vi "AcquisitionMVF_Reentrent.vi"(1 "cam conneced":bool, 4 "Numeric":i32, 5 "fake image type":enum16{"moving", "picture", "noise"}(ring), 6 "error in":errorcluster, 7 "Session":T2, 9 "Image Rev":T1) -> (0 "camera error":errorcluster, 2 "Image Dst Out":T1, 3 "Acquisition OK?":bool, 8 "time":u32)   [LabVIEW 2011]
uses:
  IMAQ Image.ctl
  IMAQdx.ctl
  NI_Vision_Development_Module.lvlib
  NI_Vision_Acquisition_Software.lvlib
  NI_AALBase.lvlib
panel:
  out "Image Out":T1
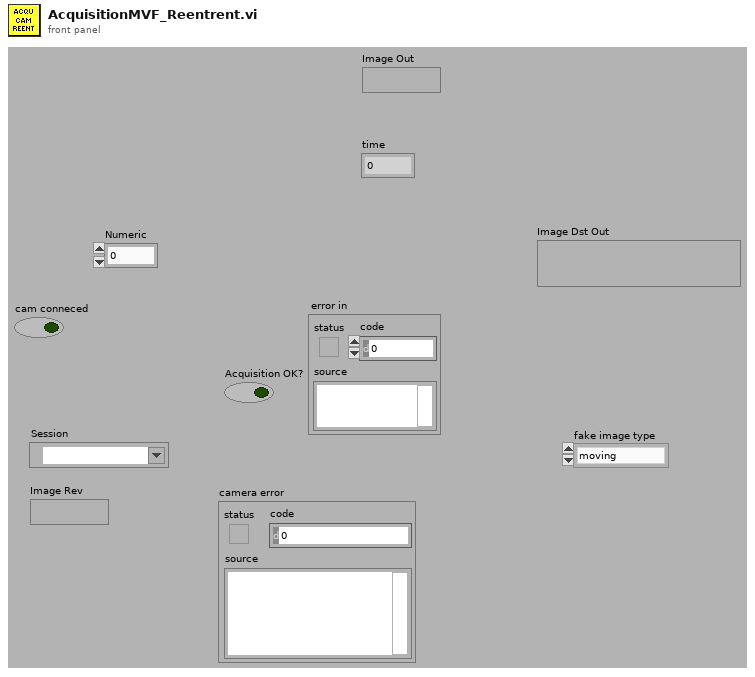
[diagram p1: front panel]
types:
  T1 = typedef "IMAQ Image.ctl" = refnum<image>
  T2 = typedef "IMAQdx.ctl" = refnum<k21>
  T3 = cluster{"Desired Font (Application)":enum16{"User-specified Font", "Application Font", "System Font", "Dialog Font"}, "[User-specified Font]":cluster{"Font Name":string, "Size":i16, "Strikeout?":bool, "Italic?":bool, "Underline?":bool, "Outline?":bool, "Shadow?":bool, "Bold?":bool, "Rotation Angle":dbl}, "Horizontal Alignment":i16, "Vertical Alignment":i16}
  T4 = typedef "Image Type" = u32
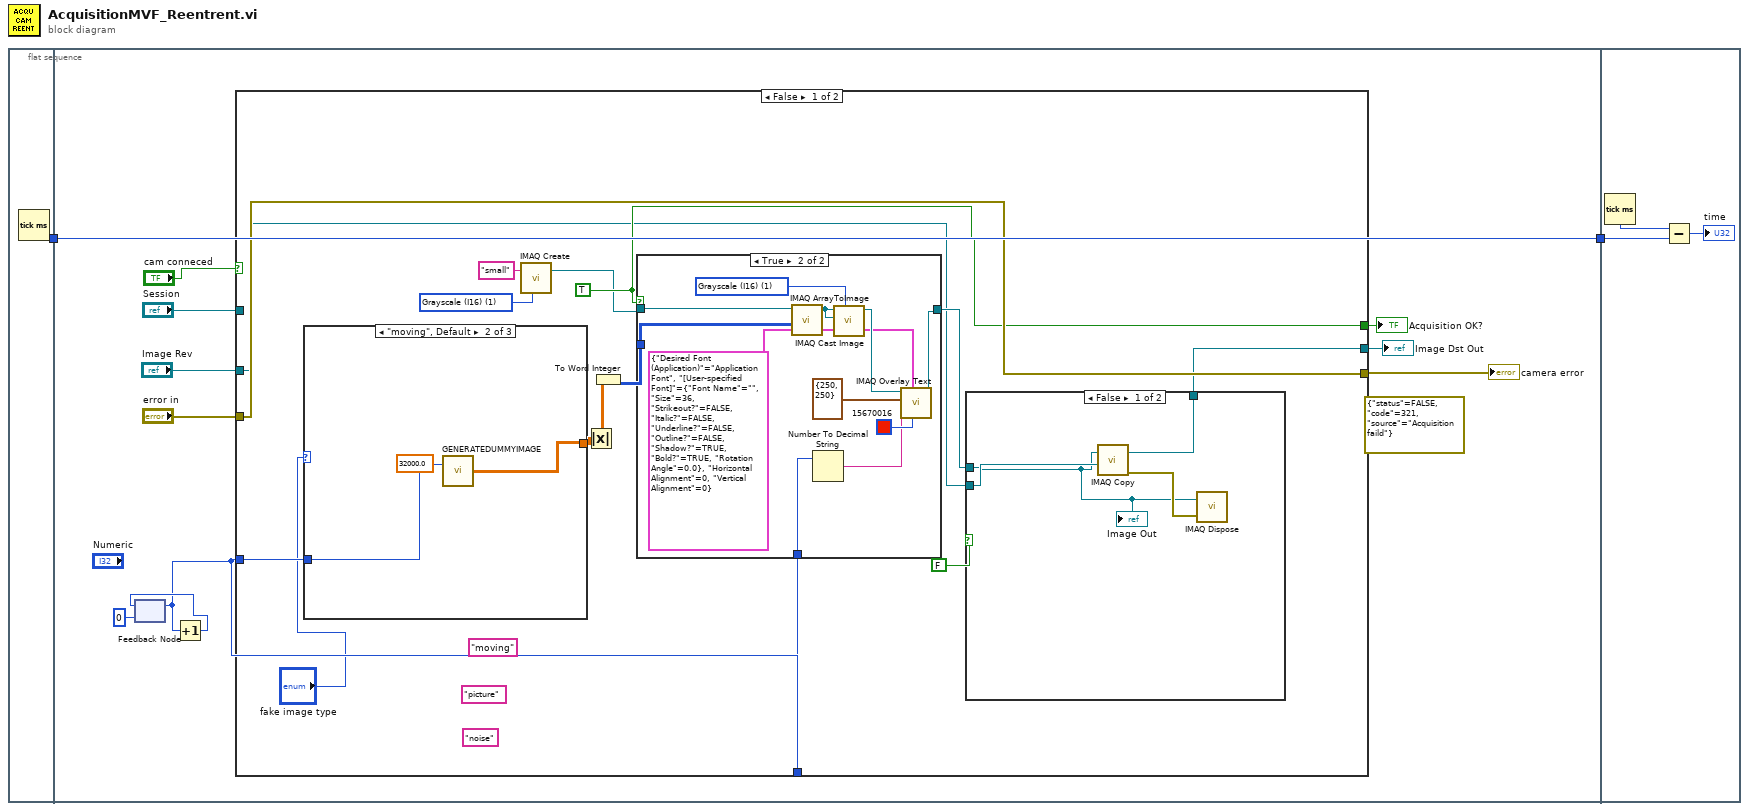
[diagram p0: block diagram]
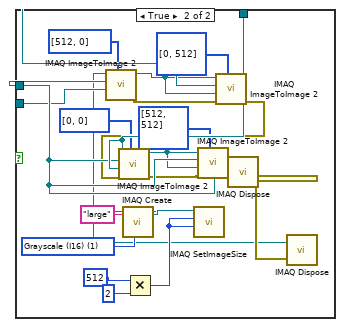
[diagram p2: hidden frame]
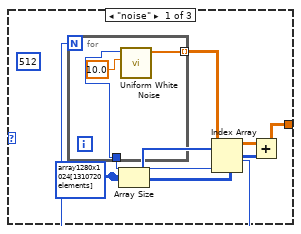
[diagram p4: hidden frame]
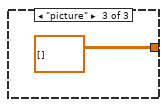
[diagram p5: hidden frame]
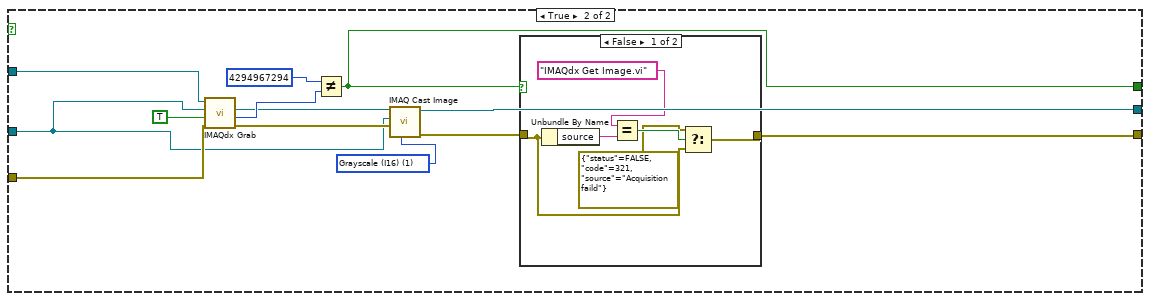
[diagram p6: hidden frame]
diagram:
  n1 = flat-sequence {
    tunnel: [w3] -> w2
    tunnel: w2 -> [w4]
    tunnel: [w4] -> w1
    tunnel: w1 -> [w101]
    frame #0 {
      n2 = Tick Count (ms)() -> (millisecond timer value=w3:u32)
    }
    frame #1 {
      (unwired) errorcluster {"status"=FALSE, "code"=321, "source"="Acquisition faild"} ("error in")
      n3 = feedback #1(0) -> (w6:i32)
      n4 = Increment(x=w6) -> (x+1=w7:i32)
      n5 = feedback-in #1(w7) -> ()
      n6 = case shown="False" "cam conneced" {
        tunnel: [w24 w81] -> w14
        tunnel: "Image Rev" -> [w19 w80]
        tunnel: "Session" -> [_ w89]
        tunnel: [w21 w86] -> w9
        tunnel: "error in" -> [w26 w85]
        tunnel: [w26 w82] -> w5
        tunnel: w6 -> [w23 _]
        tunnel: w6 -> [w25 _]
        frame False {
          w17 = T4 1 items=["Grayscale (U8)", "Grayscale (I16)", "Grayscale (SGL)", "Complex (CSG)", "RGB (U32)", "HSL (U32)", "RGB (U64)", "Grayscale (U16)"] ("Image Type")
          w24 = TRUE
          (unwired) "moving"
          (unwired) "noise"
          (unwired) "picture"
          n7 = case shown="\"moving\", Default" "fake image type" {
            tunnel: [w68 w77 dbl[][] []] -> w28
            tunnel: w23 -> [_ w78 _]
            frame "noise" {
              (unwired) 512 ("samples")
              w69 = u8[][] array1280x1024[1310720 elements] ("Image Pixels (U8) 3")
              n8 = Array Size(array=w69) -> (size(s)=w72:i32[])
              n9 = Index Array(array=w72) -> (element #1=w67:i32, element #2=w71:i32)  [unwired: 2 in]
              n10 = for {
                N: w67 -> [_]
                tunnel: [w73] -> w70 mode=indexing
                tunnel: w71 -> [w74]
                n11 = call "Uniform White Noise.vi"("amplitude"=10.0, "samples"=w74) -> ("uniform white noise"=w73:dbl[])  [unwired: 8 in, 1 out]
              }
              n12 = Add(x=w70, y=w69) -> (x+y=w68:dbl[][])
            }
            frame "moving", Default {
              n13 = call "GENERATEDUMMYIMAGE.vi"("Numeric"=w78, "amplitude"=32000.0) -> ("Gaussian Monopulse"=w77:dbl[][])
            }
            frame "picture" {
            }
          }
          n14 = call "IMAQ Create"("Image Name"="small", "Image Type"=w17) -> ("New Image"=w22:T1)  [unwired: 3 in, 1 out]
          n15 = Absolute Value(x=w28) -> (abs(x)=w29:dbl[][])
          n16 = To Word Integer(number=w29) -> (16bit integer=w27:i16[][])
          n17 = case shown="True" w24 {
            tunnel: w22 -> [w55 w57]
            tunnel: w27 -> [_ w65]
            tunnel: [w55 w60] -> w20
            tunnel: w25 -> [_ w58]
            frame False {
            }
            frame True {
              w66 = T4 1 items=["Grayscale (U8)", "Grayscale (I16)", "Grayscale (SGL)", "Complex (CSG)", "RGB (U32)", "HSL (U32)", "RGB (U64)", "Grayscale (U16)"] ("Image Type")
              n18 = call "IMAQ ArrayToImage"("Image Pixels (I16)"=w65, "Image"=w57) -> ("Image Out"=w56:T1)  [unwired: 8 in, 1 out]
              n19 = Number To Decimal String(number=w58) -> (decimal integer string=w63:string)  [unwired: 1 in]
              n20 = call "IMAQ Cast Image"("Image Type"=w66, "Image Dst"=w56, "Image Src"=w56) -> ("Image Dst Out"=w61:T1)  [unwired: 7 in, 1 out]
              n21 = call "IMAQ Overlay Text"("Text Color (black)"=u32 15670016, "Font, Size & Style"=T3 {"Desired Font (Application)"=enum."Application Font", "[User-specified Font]"={"Font Name"="", "Size"=36, "Strikeout?"=FALSE, "Italic?"=FALSE, "Underline?"=FALSE, "Outline?"=FALSE, "Shadow?"=TRUE, "Bold?"=TRUE, "Rotation Angle"=0.0}, "Horizontal Alignment"=0, "Vertical Alignment"=0}, "String"=w63, "Origin"=cluster{"X":i32, "Y":i32} {"X"=250, "Y"=250}, "Image"=w61) -> ("Image Out"=w60:T1)  [unwired: 5 in, 1 out]
            }
          }
          n22 = case shown="False" FALSE {
            tunnel: [w32 w54] -> w21
            tunnel: w20 -> [w30 w53]
            tunnel: w19 -> [w33 w52]
            frame False {
              n23 = call "IMAQ Copy"("Image Dst"=w33, "Image Src"=w30) -> ("error out"=w31:errorcluster, "Image Dst Out"=w32:T1)  [unwired: 4 in]
              n24 = call "IMAQ Dispose"("Image"=w30, "error in (no error)"=w31) -> ()  [unwired: 4 in, 1 out]
              "Image Out" <- w30
            }
            frame True {
              w51 = T4 1 items=["Grayscale (U8)", "Grayscale (I16)", "Grayscale (SGL)", "Complex (CSG)", "RGB (U32)", "HSL (U32)", "RGB (U64)", "Grayscale (U16)"] ("Image Type")
              n25 = call "IMAQ Create"("Image Name"="large", "Image Type"=w51) -> ("New Image"=w49:T1)  [unwired: 3 in, 1 out]
              n26 = Multiply(x=512, y=2) -> (x*y=w46:i32)
              n27 = call "IMAQ SetImageSize"("Y Resolution"=w46, "X Resolution"=w46, "Image"=w49) -> ("Image Out"=w43:T1)  [unwired: 2 in, 1 out]
              n28 = call "IMAQ ImageToImage 2"("Offset Left/Top"=i32[] [512, 0], "Image Dst"=w52, "Image Src (Small)"=w53, "Image Src (Large)"=w43) -> ("error out"=w40:errorcluster, "Image Dst Out"=w42:T1)  [unwired: 6 in]
              n29 = call "IMAQ ImageToImage 2"("Offset Left/Top"=i32[] [0, 512], "error in (no error)"=w40, "Image Dst"=w42, "Image Src (Small)"=w53, "Image Src (Large)"=w42) -> ("error out"=w39:errorcluster, "Image Dst Out"=w54:T1)  [unwired: 5 in]
              n30 = call "IMAQ ImageToImage 2"("Offset Left/Top"=i32[] [0, 0], "error in (no error)"=w39, "Image Dst"=w54, "Image Src (Small)"=w53, "Image Src (Large)"=w54) -> ("error out"=w38:errorcluster, "Image Dst Out"=w36:T1)  [unwired: 5 in]
              n31 = call "IMAQ ImageToImage 2"("Offset Left/Top"=i32[] [512, 512], "error in (no error)"=w38, "Image Dst"=w36, "Image Src (Small)"=w53, "Image Src (Large)"=w36) -> ("error out"=w37:errorcluster)  [unwired: 5 in, 1 out]
              n32 = call "IMAQ Dispose"("Image"=w53, "error in (no error)"=w37) -> ("error out"=w44:errorcluster)  [unwired: 4 in]
              n33 = call "IMAQ Dispose"("Image"=w43, "error in (no error)"=w44) -> ()  [unwired: 4 in, 1 out]
            }
          }
        }
        frame True {
          w88 = T4 1 items=["Grayscale (U8)", "Grayscale (I16)", "Grayscale (SGL)", "Complex (CSG)", "RGB (U32)", "HSL (U32)", "RGB (U64)", "Grayscale (U16)"] ("Image Type")
          n34 = call "IMAQdx Grab.vi"("error in"=w85, "Wait for Next Buffer? (Yes)"=TRUE, "Image In"=w80, "Session In"=w89) -> ("error out"=w84:errorcluster, "Buffer Number Out"=w91:u32, "Image Out"=w90:T1)  [unwired: 5 out]
          n35 = Not Equal?(x=u32 4294967294 ("Buffer Number Out"), y=w91) -> (x != y?=w81:bool)
          n36 = call "IMAQ Cast Image"("Image Type"=w88, "error in (no error)"=w84, "Image Dst"=w80, "Image Src"=w90) -> ("error out"=w83:errorcluster, "Image Dst Out"=w86:T1)  [unwired: 6 in]
          n37 = case shown="False" w81 {
            tunnel: w83 -> [w94 w99]
            tunnel: [w93 w99] -> w82
            frame False {
              n38 = Unbundle By Name(w94) -> ("source"=w98:string)
              n39 = Equal?(x="IMAQdx Get Image.vi", y=w98) -> (x = y?=w96:bool)
              n40 = Select(t=errorcluster {"status"=FALSE, "code"=321, "source"="Acquisition faild"} ("error in"), s=w96, f=w94) -> (s? t:f=w93:errorcluster)
            }
            frame True {
            }
          }
        }
      }
      "Acquisition OK?" <- w14
      "camera error" <- w5
      "Image Dst Out" <- w9
    }
    frame #2 {
      n41 = Tick Count (ms)() -> (millisecond timer value=w102:u32)
      n42 = Subtract(x=w102, y=w101) -> (x-y=→"time":u32)
    }
  }
